vi "All-In-One_EIC-DIRC_DAQ_v3.vi"() -> ()   [LabVIEW 2024]
uses:
  C:/Users/hpDIRC/Desktop/eic_dirc_daq-LabVIEW_new/Thorlabs/Thorlabs.MotionControl.Controls.dll
  Thorlabs/Thorlabs.MotionControl.Controls.dll
  <vilib>/numeric/Random Number (Range) DBL.vi
  C:/Users/hpDIRC/Desktop/eic_dirc_daq-LabVIEW_new/Thorlabs/Thorlabs.MotionControl.IntegratedStepperMotorsCLI.dll
  Thorlabs/Thorlabs.MotionControl.IntegratedStepperMotorsCLI.dll
  C:/Users/hpDIRC/Desktop/eic_dirc_daq-LabVIEW_new/Thorlabs/Thorlabs.MotionControl.Benchtop.StepperMotorCLI.dll
  Thorlabs/Thorlabs.MotionControl.Benchtop.StepperMotorCLI.dll
panel:
  out "Just-Measure-Last":bool
  in  "Just Measure Length":dbl=100.0
  out "counter":dbl=184.0 caption="Measurements Recorded" format="%#_13g"
  in  "Just Measure":bool
  in  "alignment points":dbl=20.0 format="%#_13g"
  in  "BA step size":dbl=0.1 format="%#_13g"
  in  "BA3 BarY start":dbl=20.0 format="%#_13g"
  in  "BA3 BarX start":dbl=229.0 format="%#_13g"
  in  "BA2 BarY start":dbl=15.0 format="%#_13g"
  in  "BA2 BarX start":dbl=229.0 format="%#_13g"
  in  "BA PDA":dbl=180.0 format="%#_13g"
  in  "BA BMA":dbl=45.0 format="%#_13g"
  in  "BA PDY":dbl=126.0 format="%#_13g"
  in  "BA PDX":dbl=268.0 format="%#_13g"
  in  "BA1 Bar Y start":dbl=30.0 format="%#_13g"
  in  "BA1 BarX start":dbl=229.0 format="%#_13g"
  in  "# BA measurement points":i32=10
  in  "# IR measurement points":i32=10
  in  "IR step size":dbl=0.1 format="%#_13g"
  in  "IR3 BarY start":dbl=32.0 format="%#_13g"
  in  "IR3 BarX start":dbl=82.5 format="%#_13g"
  in  "IR2 BarY start":dbl=15.0 format="%#_13g"
  in  "IR2 BarX start":dbl=82.5 format="%#_13g"
  in  "PB PDA":dbl=180.0 format="%#_13g"
  in  "PB BMA":dbl=45.0 format="%#_13g"
  in  "PB PDY":dbl=126.0 format="%#_13g"
  in  "PB PDX":dbl=266.0 format="%#_13g"
  in  "IR PDA":dbl=238.0 format="%#_13g"
  in  "IR BMA":dbl=17.148 format="%#_13g"
  in  "IR PDY":dbl=119.5 format="%#_13g"
  in  "IR PDX":dbl=232.0 format="%#_13g"
  in  "PB Bar Y":dbl=30.0 format="%#_13g"
  in  "PB Bar X":dbl=170.0 format="%#_13g"
  in  "IR1 Bar Y start":dbl=20.0 format="%#_13g"
  in  "IR1 Bar X start":dbl=82.5 format="%#_13g"
  out "Ambient Temperature":dbl format="%#.2g"
  in  "bar-note":u16(ring) items=["Pure Beam (PB)", "Internal Reflection (IR)", "Bulk Attenuation (BA)"]
  out "meter-error":errorcluster
  out "NM-pts-tested":dbl caption="# Pts Tested for Alignment"
  in  "align-only":bool
  in  "run-BA":bool
  in  "run-IR":bool
  in  "PDY start":dbl=105.8
  in  "PDX start":dbl=265.0
  out "run time (min)":dbl
  out "alignment-counter":dbl=184.0 format="%#_13g"
  out "Optimized Location":dbl[](array[numeric])
  in  "Test Start Delay (s)":dbl=30.0
  out "queue-length":i32 caption="Queue Elements Remaining:"
  out "next-state-cluster-const":T1={"next-state"="", "bypass-confirm"=FALSE, "PDX"=300.0, "PDY"=150.0, "BarX"=300.0, "BarY"=150.0, "BMA"=45.0, "PDA"=85.0, "bar-note"=0, "meas#"=0}
  in  "X start":dbl=262.0
  in  "X end":dbl=263.0
  in  "Y end":dbl=121.5 format="%#_13g"
  in  "X step size":dbl=0.2 format="%#_13g"
  in  "Y step size":dbl=0.2
  in  "Y start":dbl=120.5 format="%#_13g"
  in  "centered-diode-scan":bool
  out "keep-file":bool
  out "main-stage-refs":T2
  out "state-queue":T3(array[cluster])
  out "loop-rate":u32
  out "meter-stat":bool caption="Log Status"
  out "stage-stat":bool caption="Log Status"
  out "Current Time:":string
  out "log-error":errorcluster
  out "log-path":path caption="Path Data Will Save To:"
  out "start-msg":string
  out "stage-error":errorcluster
  in  "PD Angle":refnum<k24>(container)
  in  "Brewster":refnum<k24>(container)
  in  "PD Y":refnum<k24>(container)
  in  "PD X":refnum<k24>(container)
  in  "BAR Y":refnum<k24>(container)
  in  "stop":bool
  in  "BAR X":refnum<k24>(container)
  out "pd-plt":cluster{"[0]":dbl, "[1]":dbl, "[2]":dbl}(graph) caption="Measurement History"
  out "pd3_v":dbl caption="PD 3" format="%#.4g"
  out "pd2_v":dbl caption="PD 2" format="%#.4g"
  out "pd1_v":dbl caption="PD 1" format="%#.4g"
  # "IR settings"
  # "°C"
  # "EXPERT DEBUGGING INFO"
  # "A"
  # "A"
  # "BA settings"
  # "A"
  # "Work In Progress - please do not use"
  # "Bar Note Readback:"
  # "PB settings"
  # "PD ONLY SCAN - CENTERED"
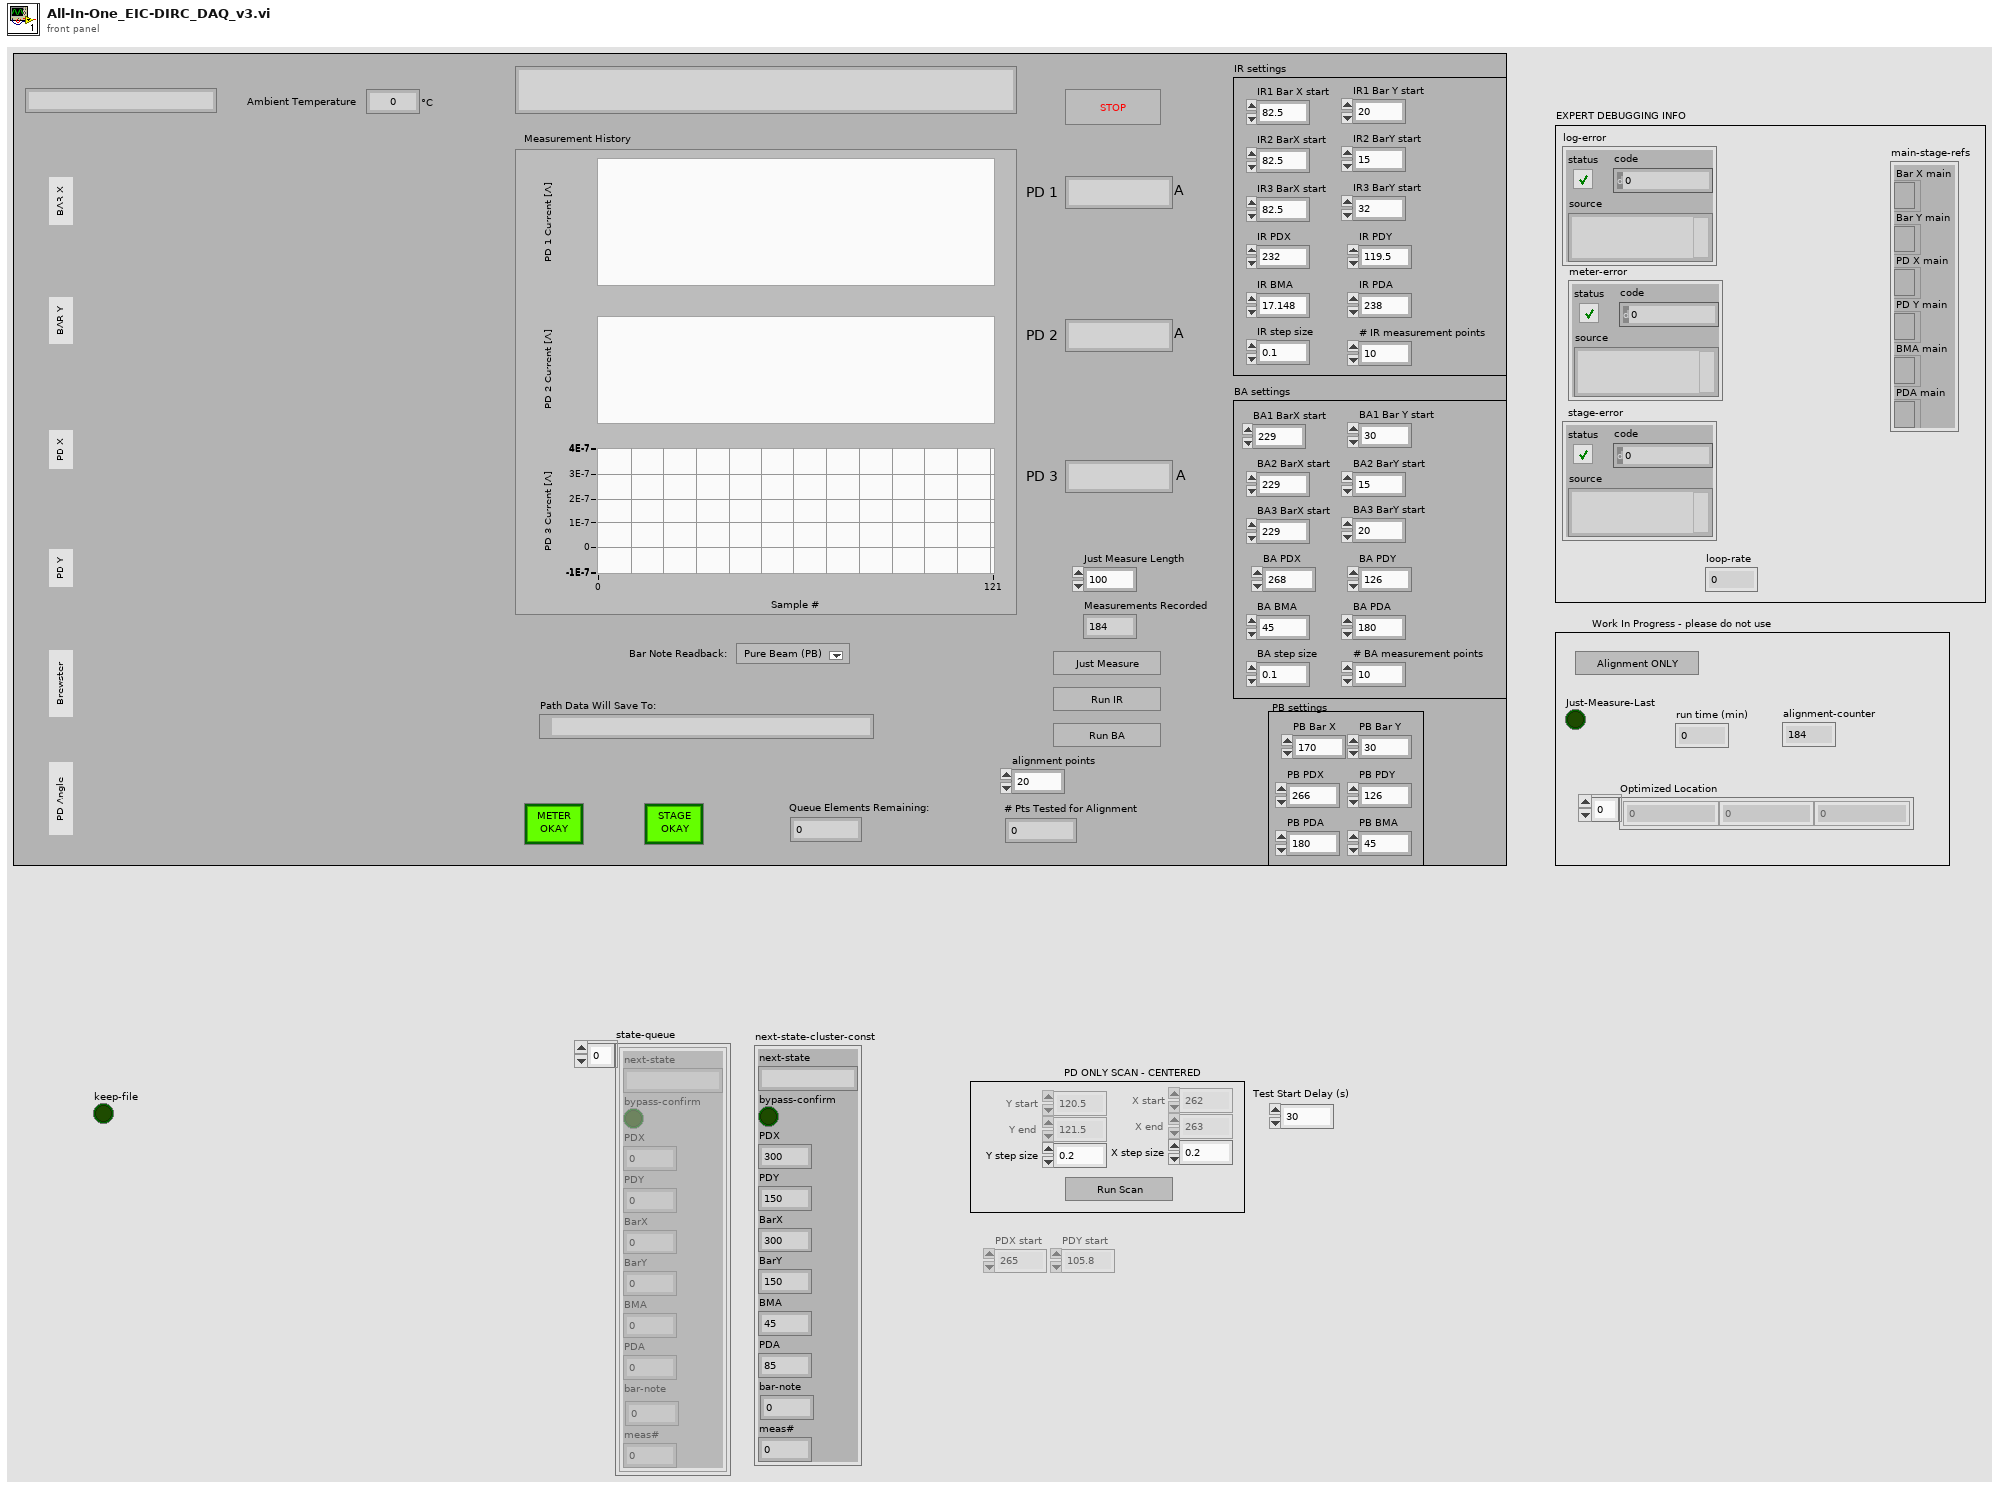
[diagram p1: front panel]
types:
  T1 = cluster{"next-state":string, "bypass-confirm":bool, "PDX":dbl, "PDY":dbl, "BarX":dbl, "BarY":dbl, "BMA":dbl, "PDA":dbl, "bar-note":u8, "meas#":u32}
  T2 = cluster{"Bar X main":refnum<k24>, "Bar Y main":refnum<k24>, "PD X main":refnum<k24>, "PD Y main":refnum<k24>, "BMA main":refnum<k24>, "PDA main":refnum<k24>}
  T3 = cluster{"next-state":string, "bypass-confirm":bool, "PDX":dbl, "PDY":dbl, "BarX":dbl, "BarY":dbl, "BMA":dbl, "PDA":dbl, "bar-note":u8, "meas#":u32}[]
  T4 = cluster{"Bar X":refnum<k24>, "Bar Y":refnum<k24>, "PD X":refnum<k24>, "PD Y":refnum<k24>, "Brewster":refnum<k24>, "PD Angle":refnum<k24>}
  T5 = enum16{"open", "replace", "create", "open or create", "replace or create", "replace or create with confirmation"}
  T6 = cluster{"alpha":dbl, "gamma":dbl, "rho":dbl, "sigma":dbl, "simplex L":dbl}
  T7 = cluster{"next-state":string, "mode-select":enum32{"IR", "Pure", "Bulk", "Bar Out", "stored-loc", "custom"}, "bypass-confirm":bool, "PDX":dbl, "PDY":dbl, "BarX":dbl, "BarY":dbl, "BMA":dbl, "PDA":dbl, "bar-note":bool}
  T8 = cluster{"[0]":dbl, "[1]":dbl, "[2]":dbl, "[3]":dbl, "[4]":dbl, "[5]":dbl, "[6]":dbl, "[7]":dbl, "[8]":dbl}
  T9 = cluster{"Bar X":dbl, "Bar Y":dbl, "PD X":dbl, "PD Y":dbl, "BMA":dbl, "PDA":dbl}
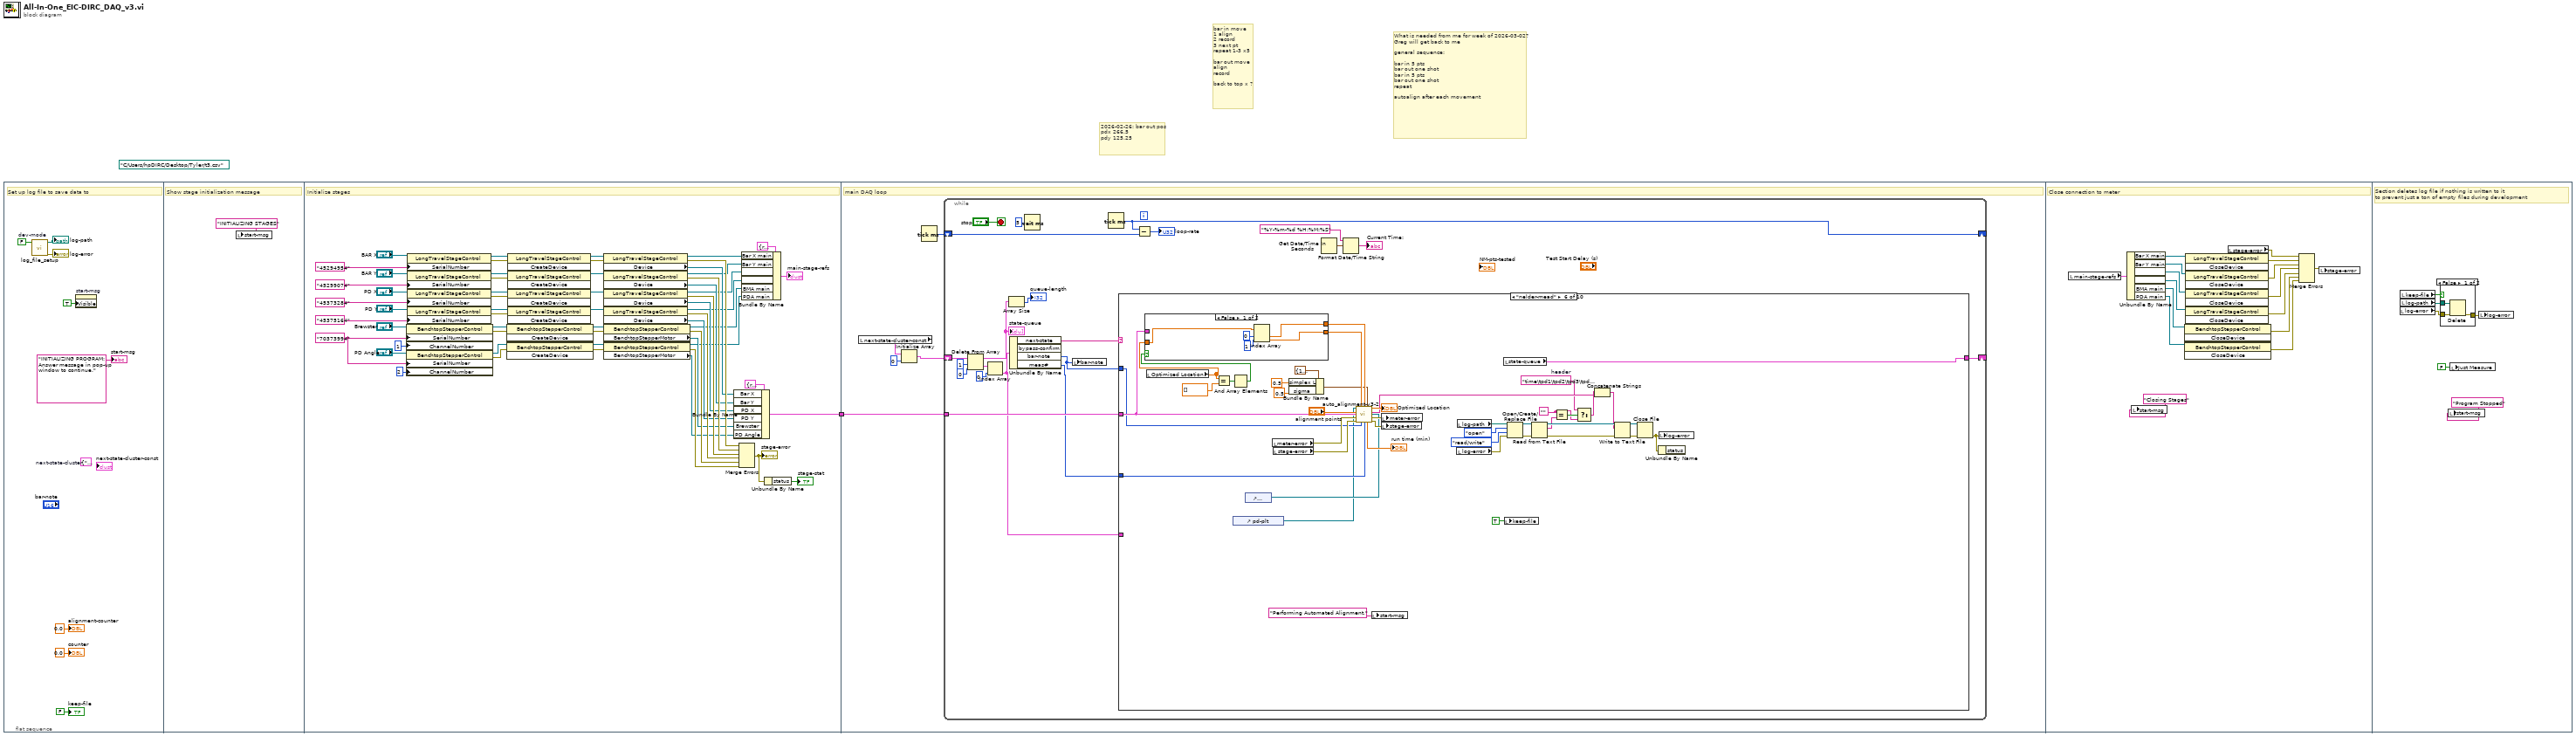
[diagram p0: block diagram]
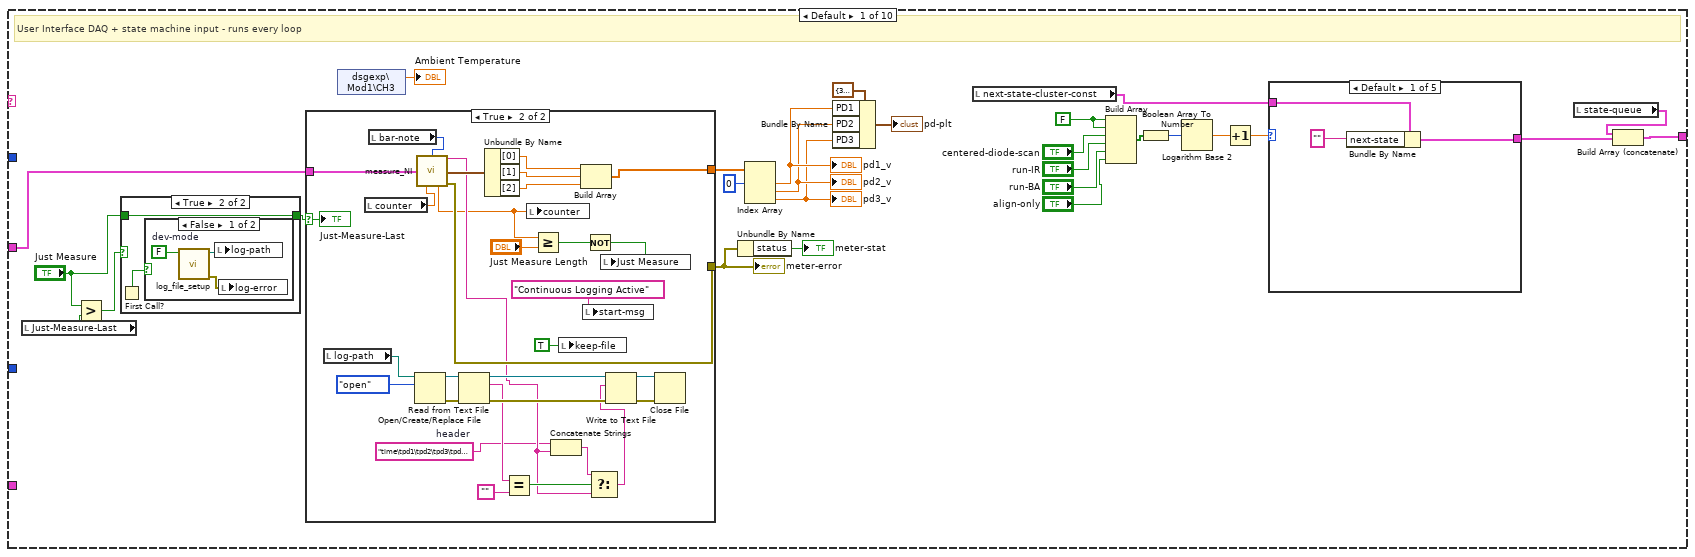
[diagram p2: hidden frame]
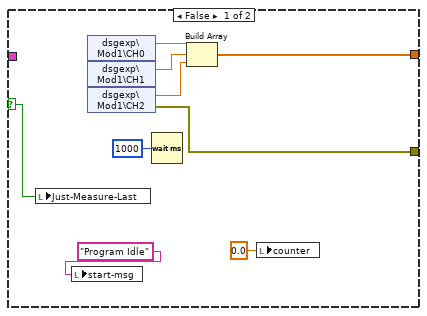
[diagram p5: hidden frame]
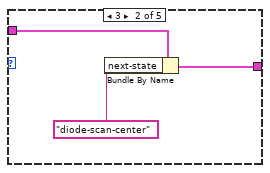
[diagram p6: hidden frame]
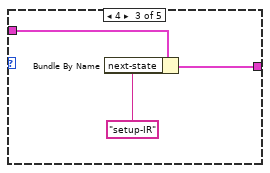
[diagram p7: hidden frame]
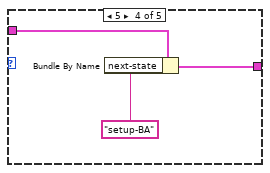
[diagram p8: hidden frame]
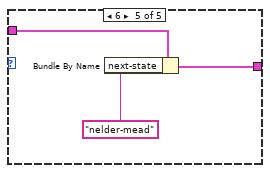
[diagram p9: hidden frame]
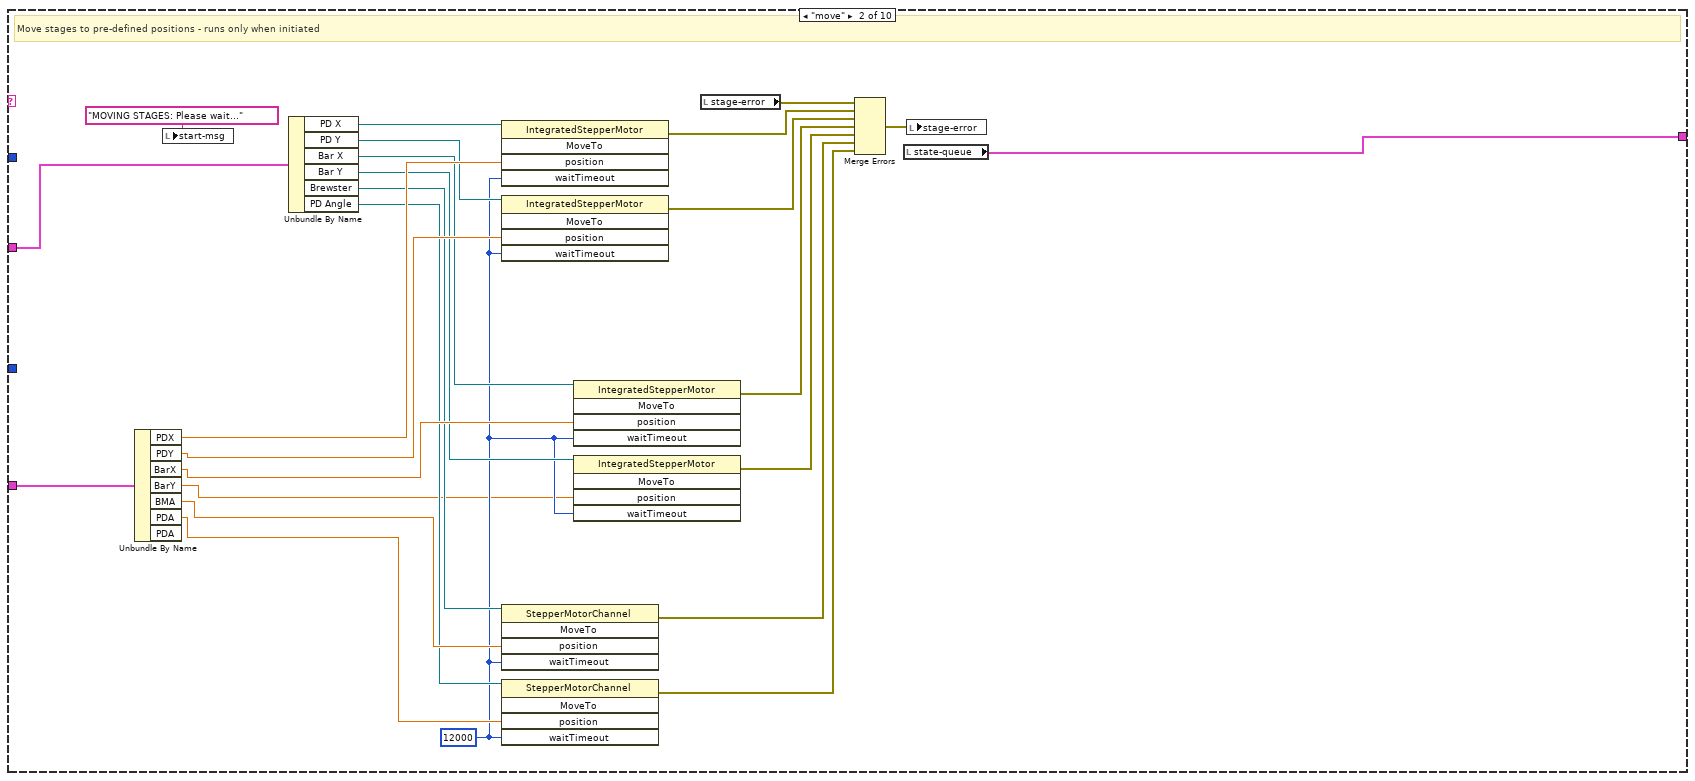
[diagram p10: hidden frame]
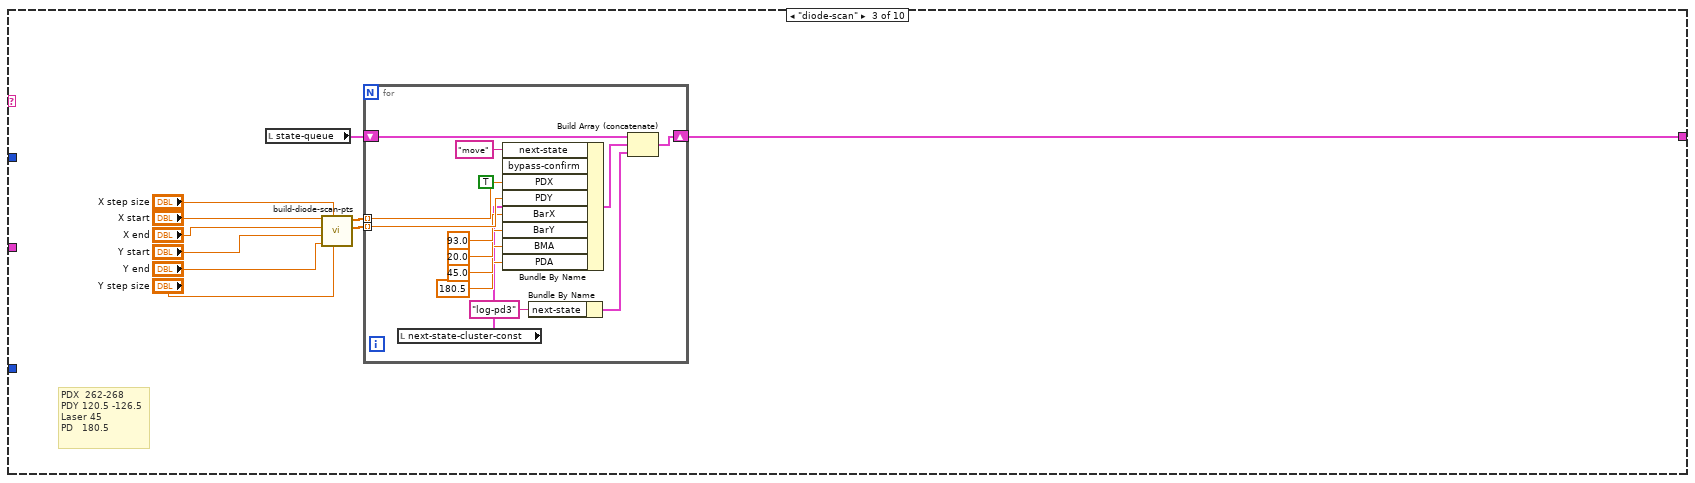
[diagram p11: hidden frame]
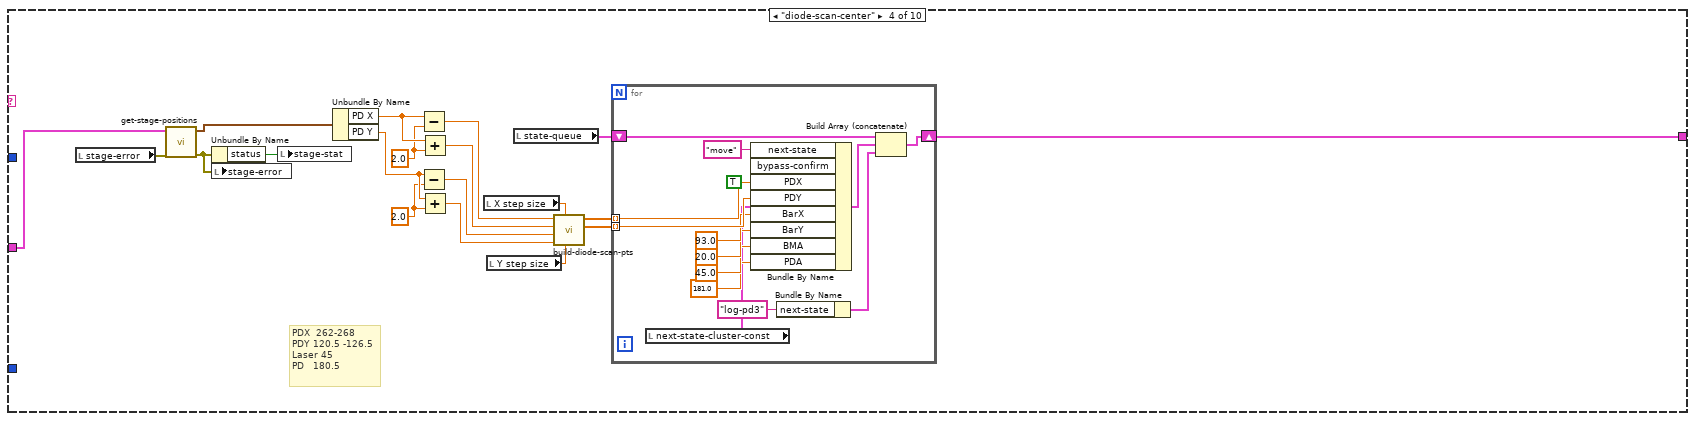
[diagram p12: hidden frame]
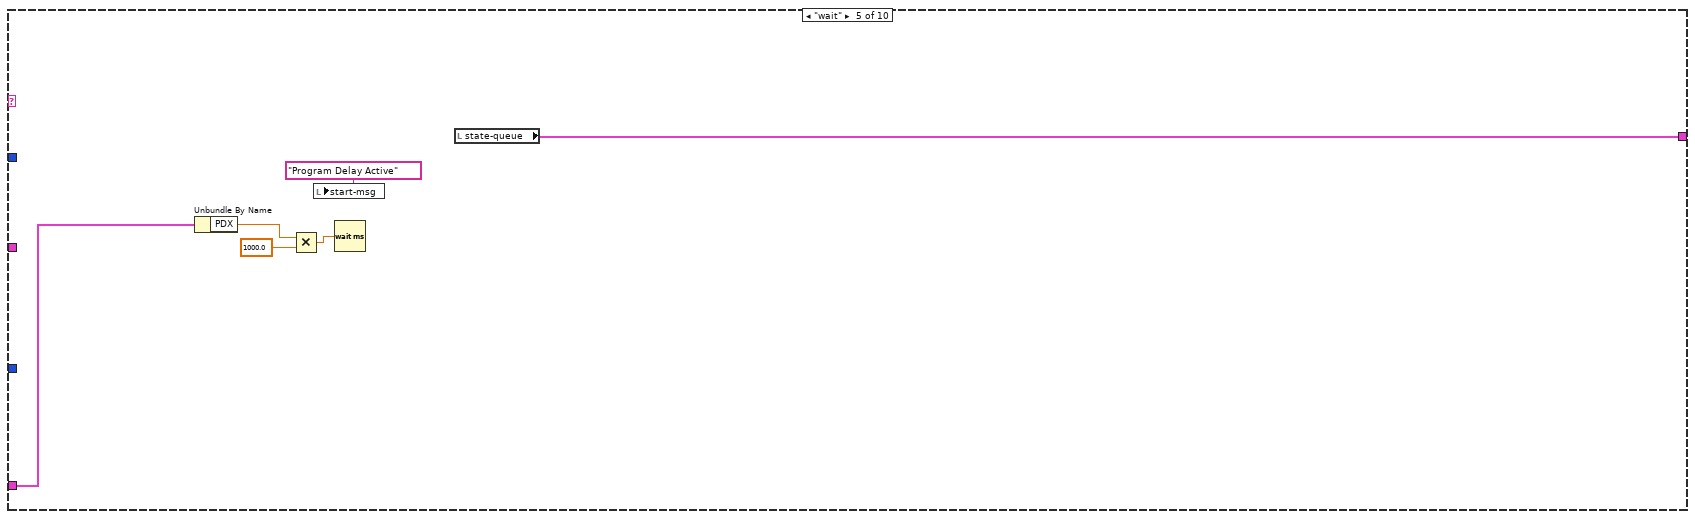
[diagram p13: hidden frame]
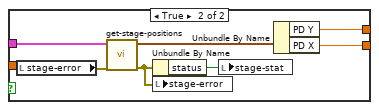
[diagram p14: hidden frame]
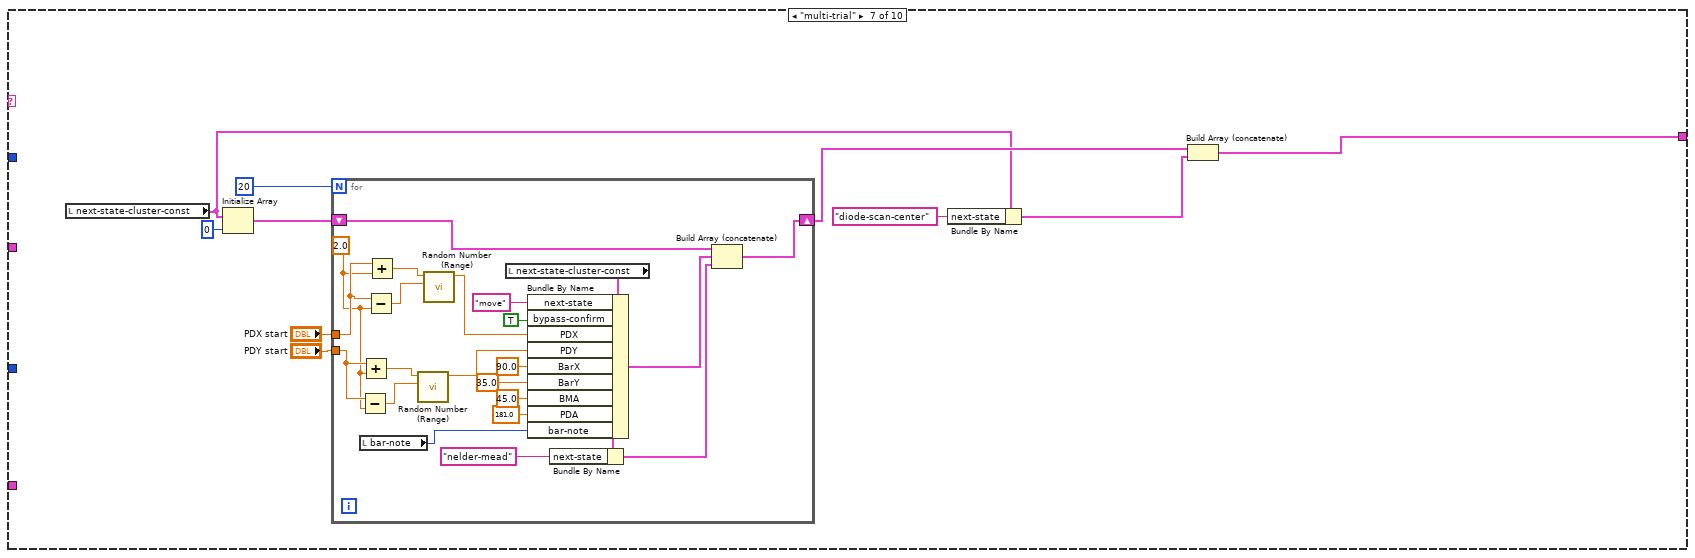
[diagram p15: hidden frame]
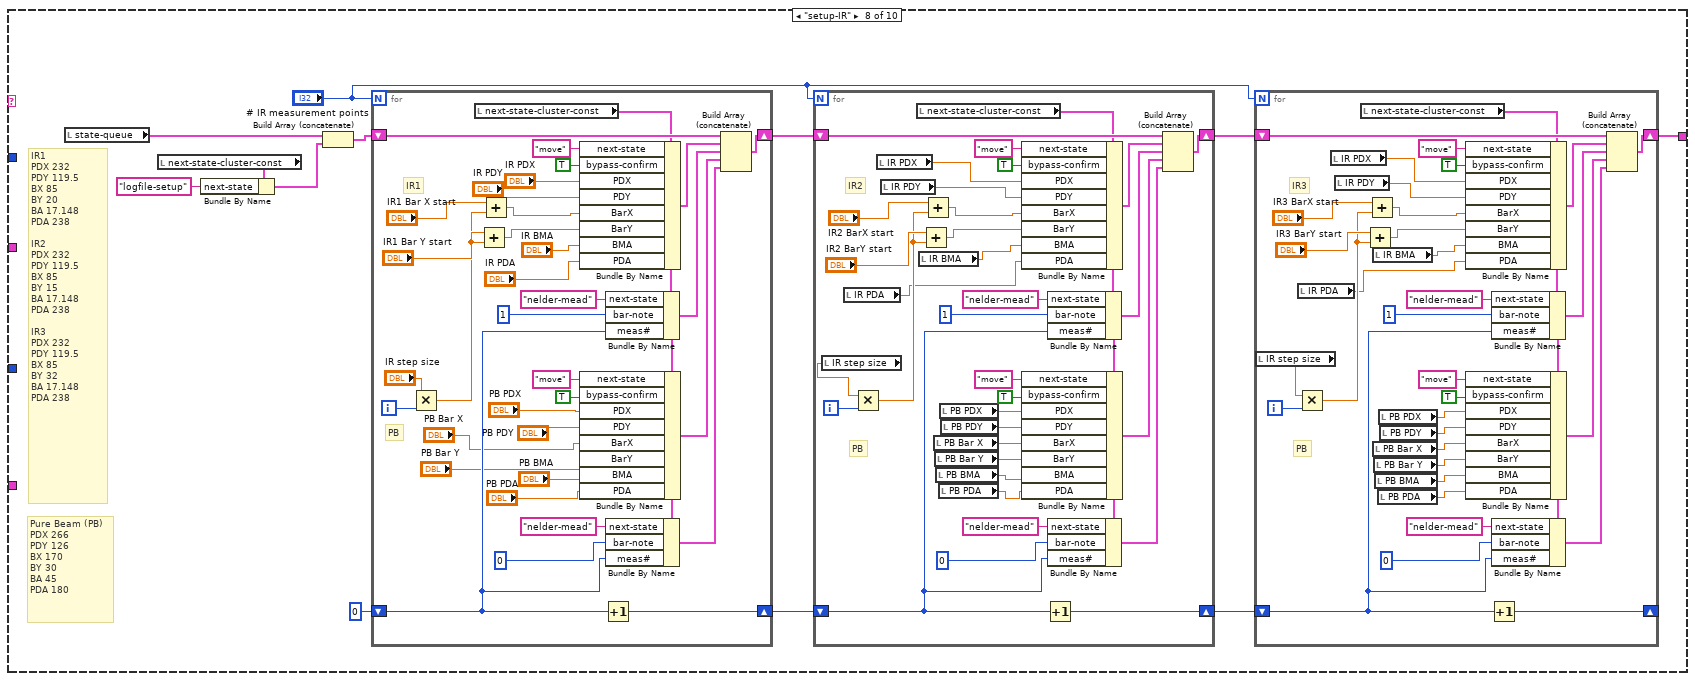
[diagram p16: hidden frame]
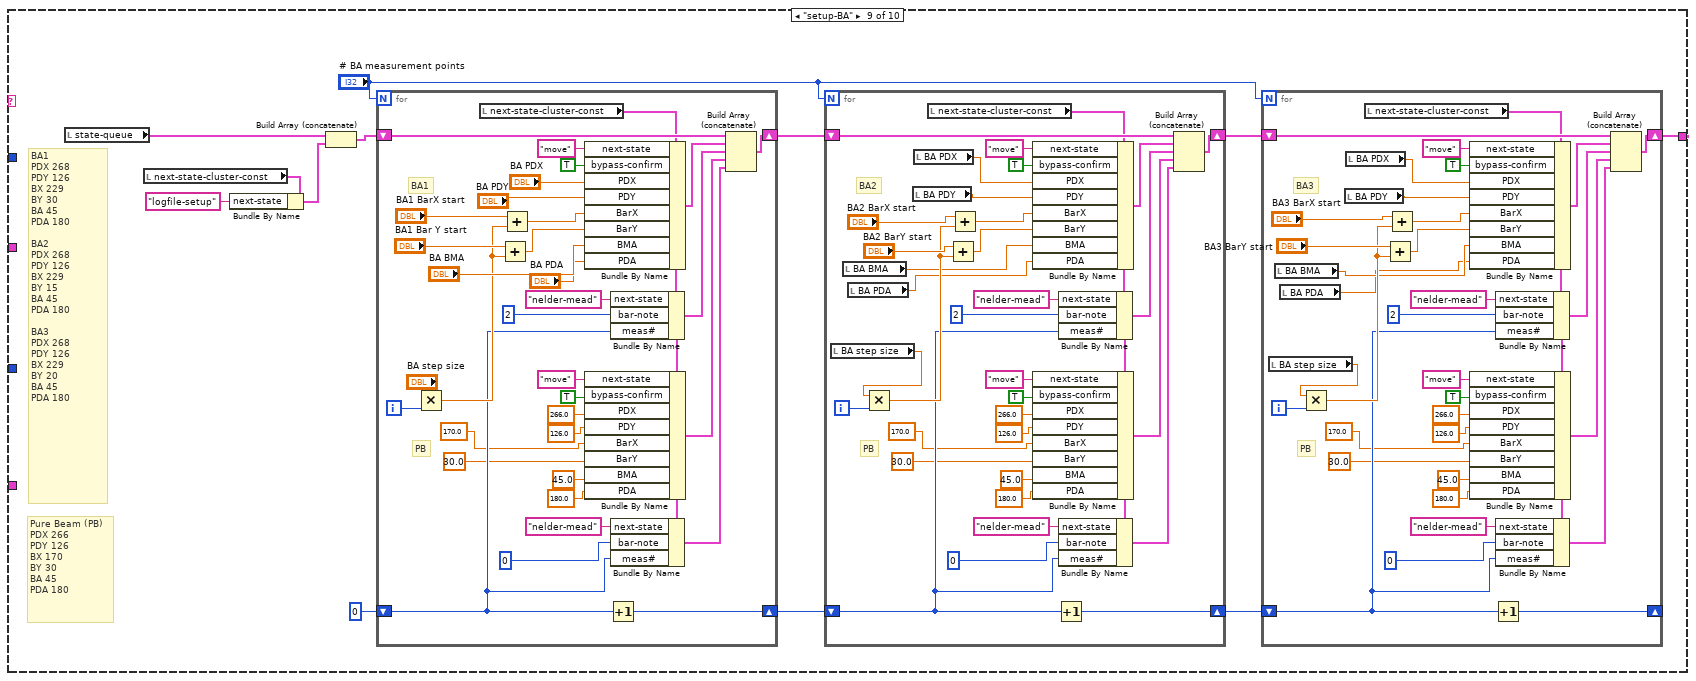
[diagram p17: hidden frame]
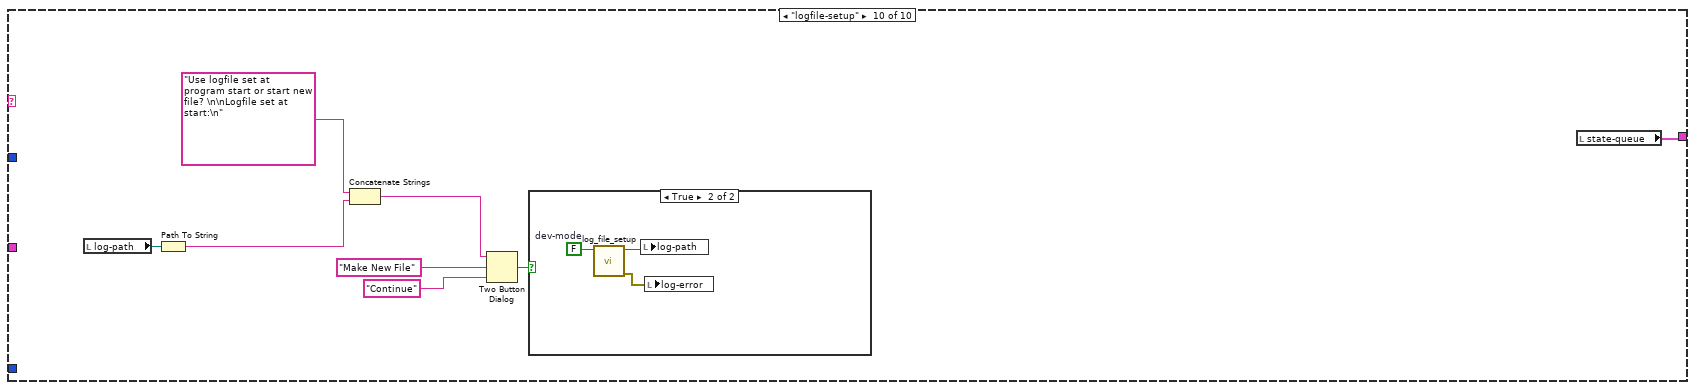
[diagram p18: hidden frame]
diagram:
  (unwired) path "C:/Users/hpDIRC/Desktop/Tyler/t3.csv" ("log-path")
  # "2026-02-26: bar out pos\npdx 266.5\npdy 125.25"
  # "bar in move\n1 align\n2 record\n3 next pt\nrepeat 1-3 x5\n\nbar out move\nalign\nrecord\n\nback to top x ?"
  # "What is needed from me for week of 2026-03-02?\nGreg will get back to me\n\ngeneral sequence:\n\nbar in 5 pts \nbar out one shot\nbar in 5 pts\nbar out one shot\nrepeat\n\nautoalign after each movement"
  n1 = flat-sequence {
    tunnel: [w21] -> w1
    tunnel: w1 -> [w72]
    frame #0 {
      w5 = FALSE  # dev-mode
      (unwired) T7 {"next-state"="", "mode-select"=enum."IR", "bypass-confirm"=FALSE, "PDX"=300.0, "PDY"=150.0, "BarX"=300.0, "BarY"=150.0, "BMA"=45.0, "PDA"=85.0, "bar-note"=FALSE}  # next-state-cluster
      # "Set up log file to save data to"
      n2 = call "log_file_setup.vi"("dev-mode"=w5) -> ("error out"=→"log-error":errorcluster, "appended path"=→"log-path":path)  [unwired: 8 in, 1 out]
      n3 = property on="start-msg" class="Str"("Visible"=TRUE) -> ()  [unwired: 2 in, 2 out]
      "start-msg" <- "INITIALIZING PROGRAM: Answer message in pop-up window to continue." ("String")
      "keep-file" <- FALSE
      "alignment-counter" <- 0.0 ("alignment-counter")
      "counter" <- 0.0 ("alignment-counter")
    }
    frame #1 {
      # "Show stage initialization message"
      n4 = local write "start-msg"("INITIALIZING STAGES" ("String")) -> ()
    }
    frame #2 {
      w28 = "70373994" ("SerialNumber")
      # "Initialize stages"
      n5 = property class="BenchtopStepperControl"(reference="Brewster", "SerialNumber"=w28, "ChannelNumber"=1) -> (reference out=w54:refnum<k24>, error out=w55:errorcluster)  [unwired: 1 in]
      n6 = property class="BenchtopStepperControl"(reference="PD Angle", "SerialNumber"=w28, "ChannelNumber"=2) -> (reference out=w53:refnum<k24>, error out=w56:errorcluster)  [unwired: 1 in]
      n7 = property class="LongTravelStageControl"(reference="BAR X", "SerialNumber"="45294954") -> (reference out=w31:refnum<k24>, error out=w38:errorcluster)  [unwired: 1 in]
      n8 = property class="LongTravelStageControl"(reference="BAR Y", "SerialNumber"="45299074") -> (reference out=w32:refnum<k24>, error out=w39:errorcluster)  [unwired: 1 in]
      n9 = property class="LongTravelStageControl"(reference="PD X", "SerialNumber"="45373284") -> (reference out=w35:refnum<k24>, error out=w40:errorcluster)  [unwired: 1 in]
      n10 = property class="LongTravelStageControl"(reference="PD Y", "SerialNumber"="45375164") -> (reference out=w36:refnum<k24>, error out=w41:errorcluster)  [unwired: 1 in]
      n11 = invoke class="BenchtopStepperControl" method="CreateDevice"(reference=w54, error in=w55) -> (reference out=w51:refnum<k24>, error out=w49:errorcluster)  [unwired: 1 in, 1 out]
      n12 = invoke class="BenchtopStepperControl" method="CreateDevice"(reference=w53, error in=w56) -> (reference out=w50:refnum<k24>, error out=w52:errorcluster)  [unwired: 1 in, 1 out]
      n13 = invoke class="LongTravelStageControl" method="CreateDevice"(reference=w31, error in=w38) -> (reference out=w44:refnum<k24>, error out=w48:errorcluster)  [unwired: 1 in, 1 out]
      n14 = invoke class="LongTravelStageControl" method="CreateDevice"(reference=w32, error in=w39) -> (reference out=w45:refnum<k24>)  [unwired: 1 in, 2 out]
      n15 = invoke class="LongTravelStageControl" method="CreateDevice"(reference=w35, error in=w40) -> (reference out=w46:refnum<k24>)  [unwired: 1 in, 2 out]
      n16 = invoke class="LongTravelStageControl" method="CreateDevice"(reference=w36, error in=w41) -> (reference out=w47:refnum<k24>)  [unwired: 1 in, 2 out]
      n17 = property class="BenchtopStepperControl"(reference=w51, error in=w49) -> (reference out=w15:refnum<k24>, error out=w66:errorcluster, "BenchtopStepperMotor"=w61:refnum<k24>)
      n18 = property class="BenchtopStepperControl"(reference=w50, error in=w52) -> (reference out=w14:refnum<k24>, error out=w67:errorcluster, "BenchtopStepperMotor"=w62:refnum<k24>)
      n19 = property class="LongTravelStageControl"(reference=w44, error in=w48) -> (reference out=w19:refnum<k24>, error out=w68:errorcluster, "Device"=w57:refnum<k24>)
      n20 = property class="LongTravelStageControl"(reference=w45) -> (reference out=w18:refnum<k24>, error out=w63:errorcluster, "Device"=w58:refnum<k24>)  [unwired: 1 in]
      n21 = property class="LongTravelStageControl"(reference=w46) -> (reference out=w17:refnum<k24>, error out=w64:errorcluster, "Device"=w59:refnum<k24>)  [unwired: 1 in]
      n22 = property class="LongTravelStageControl"(reference=w47) -> (reference out=w16:refnum<k24>, error out=w65:errorcluster, "Device"=w60:refnum<k24>)  [unwired: 1 in]
      n23 = Bundle By Name(cluster=T4 {"Bar X"=refnum, "Bar Y"=refnum, "PD X"=refnum, "PD Y"=refnum, "Brewster"=refnum, "PD Angle"=refnum}, "Bar X"=w57, "Bar Y"=w58, "PD X"=w59, "PD Y"=w60, "Brewster"=w61, "PD Angle"=w62) -> (w21:T4)
      n24 = Merge Errors(w68, w63, w64, w65, w66, w67) -> (w12:errorcluster)
      "stage-error" <- w12
      n25 = Bundle By Name(cluster=T2 {"Bar X main"=refnum, "Bar Y main"=refnum, "PD X main"=refnum, "PD Y main"=refnum, "BMA main"=refnum, "PDA main"=refnum}, "Bar X main"=w19, "Bar Y main"=w18, "PD X main"=w17, "PD Y main"=w16, "BMA main"=w15, "PDA main"=w14) -> (→"main-stage-refs":T2)
      n26 = Unbundle By Name(w12) -> ("status"=→"stage-stat":bool)
    }
    frame #3 {
      # "main DAQ loop"
      n27 = local read "next-state-cluster-const"() -> (w69:T1)
      n28 = Initialize Array(w69, 0 ("dimension size")) -> (w71:T3)
      n29 = Tick Count (ms)() -> (millisecond timer value=w73:u32)
      n30 = while {
        shift-right: [w93] -> _
        shift-left: w73 -> [w92]
        tunnel: w72 -> [w90]
        shift-right: [w79] -> _
        shift-left: w71 -> [w81]
        stop <- "stop" stop-if-true
        n31 = Delete From Array(array=w81, length=1, index=0) -> (deleted portion=w80:T3, array with subset deleted=w77:T3)
        "state-queue" <- w77
        n32 = Index Array(array=w80, index=0) -> (element=w78:T1)
        n33 = Array Size(array=w77) -> (size(s)=→"queue-length":i32)
        n34 = Unbundle By Name(w78) -> ("next-state"=w82:string, "bar-note"=w76:u8, "meas#"=w75:u32)  [unwired: 1 out]
        n35 = Wait (ms)(milliseconds to wait=u32 5) -> ()  [unwired: 1 out]
        n36 = local write "bar-note"(w76) -> ()
        n37 = Tick Count (ms)() -> (millisecond timer value=w93:u32)
        n38 = case shown="\"nelder-mead\"" w82 {
          tunnel: w90 -> [w101 w210 _ w243 _ w302 _ _ _ _]
          tunnel: [w113 w209 w217 w250 w269 w316 w331 w366 w480 w596] -> w79
          tunnel: w78 -> [_ w207 _ _ w270 _ _ _ _ _]
          tunnel: w76 -> [_ _ _ _ _ w301 _ _ _ _]
          tunnel: w75 -> [_ _ _ _ _ w300 _ _ _ _]
          frame Default {
            w102 = FALSE ("element")
            # "User Interface DAQ + state machine input - runs every loop"
            n39 = local read "Just-Measure-Last"() -> (w98:bool)
            n40 = Greater?(x="Just Measure", y=w98) -> (0:w97:bool)
            n41 = case shown="True" w97 {
              tunnel: "Just Measure" -> [w123 w125]
              tunnel: [w123 w125] -> w95
              frame False {
              }
              frame True {
                n42 = First Call?() -> (First Call?: T/F=w124:bool)
                n43 = case shown="False" w124 {
                  frame False {
                    w126 = FALSE  # dev-mode
                    n44 = call "log_file_setup.vi"("dev-mode"=w126) -> ("error out"=w127:errorcluster, "appended path"=w128:path)  [unwired: 8 in, 1 out]
                    n45 = local write "log-path"(w128) -> ()
                    n46 = local write "log-error"(w127) -> ()
                  }
                  frame True {
                  }
                }
              }
            }
            n47 = case shown="True" w95 {
              selector: w95 -> [w130 w141]
              tunnel: [w139 w163] -> w103
              tunnel: w101 -> [_ w170]
              tunnel: [w132 w168] -> w99
              frame False {
                n48 = local write "Just-Measure-Last"(w130) -> ()
                n49 = local write "start-msg"("Program Idle" ("String")) -> ()
                n50 = shared-variable "dsgexp\\Mod1\\CH0"() -> (w138:dbl, error out=w135:errorcluster)  [unwired: 1 in]
                n51 = shared-variable "dsgexp\\Mod1\\CH1"(error in=w135) -> (w137:dbl, error out=w134:errorcluster)
                n52 = shared-variable "dsgexp\\Mod1\\CH2"(error in=w134) -> (w136:dbl, error out=w132:errorcluster)
                n53 = Wait (ms)(milliseconds to wait=u32 1000) -> ()  [unwired: 1 out]
                n54 = Build Array(w138, w137, w136) -> (w139:dbl[])
                n55 = local write "counter"(0.0 ("counter")) -> ()
              }
              frame True {
                w148 = "time\tpd1\tpd2\tpd3\tpd3/pd1\tpd2/pd1\tbx\tby\tpdx\tpdy\tpda\tbm\tbar-note\tmeas#\tpt#\n"  # header
                n56 = local read "log-path"() -> (w161:path)
                n57 = local read "counter"() -> (w162:dbl)
                n58 = local read "bar-note"() -> (w169:u16)
                n59 = Open/Create/Replace File(file path (use dialog)=w161, operation (0:open)=T5."open") -> (refnum out=w158:refnum<file>, error out=w159:errorcluster)  [unwired: 4 in, 1 out]
                n60 = call "measure_NI.vi"("bar-note"=w169, "stage-refs"=w170, "counter-in"=w162) -> ("logfile-line-out"=w149:string, "PD out"=w167:T8, "counter-out"=w145:dbl, "stage-error-out"=w168:errorcluster)  [unwired: 7 in, 2 out]
                n61 = Read from Text File(file (use dialog)=w158, error in=w159) -> (refnum out=w156:refnum<file>, text=w151:string, error out=w157:errorcluster)  [unwired: 2 in, 1 out]
                n62 = Unbundle By Name(w167) -> ("[0]"=w166:dbl, "[1]"=w165:dbl, "[2]"=w164:dbl)
                n63 = Equal?(x=w151, y="") -> (x = y?=w150:bool)
                n64 = local write "counter"(w145) -> ()
                n65 = Greater Or Equal?(x=w145, y="Just Measure Length") -> (x >= y?=w143:bool)
                n66 = Concatenate Strings(w148, w149) -> (w147:string)
                n67 = local write "keep-file"(TRUE ("keep-file")) -> ()
                n68 = Build Array(w166, w165, w164) -> (w163:dbl[])
                n69 = local write "start-msg"("Continuous Logging Active" ("String")) -> ()
                n70 = Not(x=w143) -> (.not. x?=w142:bool)
                n71 = Select(t=w147, s=w150, f=w149) -> (s? t:f=w146:string)
                n72 = local write "Just Measure"(w142) -> ()
                n73 = Write to Text File(file (use dialog)=w156, text=w146, error in=w157) -> (refnum out=w154:refnum<file>, error out=w155:errorcluster)  [unwired: 1 in, 1 out]
                n74 = Close File(refnum=w154, error in=w155) -> ()  [unwired: 2 out]
                "Just-Measure-Last" <- w141
              }
            }
            "meter-error" <- w99
            n75 = shared-variable "dsgexp\\Mod1\\CH3"() -> (→"Ambient Temperature":dbl)  [unwired: 1 in, 1 out]
            n76 = Unbundle By Name(w99) -> ("status"=→"meter-stat":bool)
            n77 = Index Array(array=w103, index #1=0 ("index")) -> (element #1=w120:dbl, element #2=w119:dbl, element #3=w118:dbl)  [unwired: 2 in]
            "pd3_v" <- w118
            "pd2_v" <- w119
            "pd1_v" <- w120
            n78 = Bundle By Name(cluster=cluster{"PD1":dbl, "PD2":dbl, "PD3":dbl} {"PD1"=3e-05, "PD2"=3e-05, "PD3"=3e-05} ("PD ranges"), "PD1"=w120, "PD2"=w119, "PD3"=w118) -> (→"pd-plt":cluster{"PD1":dbl, "PD2":dbl, "PD3":dbl})
            n79 = local read "next-state-cluster-const"() -> (w111:T1)
            n80 = Build Array(w102, w102, "centered-diode-scan", "run-IR", "run-BA", "align-only") -> (w116:bool[])
            n81 = Boolean Array To Number(Boolean array=w116) -> (number=w108:u32)
            n82 = Logarithm Base 2(1:w108) -> (0:w110:dbl)
            n83 = Increment(x=w110) -> (x+1=w109:dbl)
            n84 = case shown="Default" w109 {
              tunnel: w111 -> [w173 w176 w179 w182 w185]
              tunnel: [w171 w174 w177 w180 w183] -> w112
              frame Default {
                n85 = Bundle By Name(cluster=w173, "next-state"="") -> (w171:T1)
              }
              frame 3 {
                n86 = Bundle By Name(cluster=w176, "next-state"="diode-scan-center") -> (w174:T1)
              }
              frame 4 {
                n87 = Bundle By Name(cluster=w179, "next-state"="setup-IR") -> (w177:T1)
              }
              frame 5 {
                n88 = Bundle By Name(cluster=w182, "next-state"="setup-BA") -> (w180:T1)
              }
              frame 6 {
                n89 = Bundle By Name(cluster=w185, "next-state"="nelder-mead") -> (w183:T1)
              }
            }
            n90 = local read "state-queue"() -> (w114:T3)
            n91 = Build Array (concatenate)(w114, w112) -> (w113:T3)
          }
          frame "move" {
            w187 = 12000 ("waitTimeout")
            # "Move stages to pre-defined positions - runs only when initiated"
            n92 = Unbundle By Name(w207) -> ("PDX"=w206:dbl, "PDY"=w205:dbl, "BarX"=w204:dbl, "BarY"=w186:dbl, "BMA"=w203:dbl, "PDA"=w202:dbl)  [unwired: 1 out]
            n93 = local write "start-msg"("MOVING STAGES: Please wait..." ("String")) -> ()
            n94 = Unbundle By Name(w210) -> ("PD X"=w193:refnum<k24>, "PD Y"=w188:refnum<k24>, "Bar X"=w189:refnum<k24>, "Bar Y"=w190:refnum<k24>, "Brewster"=w191:refnum<k24>, "PD Angle"=w192:refnum<k24>)
            n95 = invoke class="IntegratedStepperMotor" method="MoveTo"(reference=w193, "position"=w206, "waitTimeout"=w187) -> (error out=w200:errorcluster)  [unwired: 2 in, 4 out]
            n96 = invoke class="IntegratedStepperMotor" method="MoveTo"(reference=w188, "position"=w205, "waitTimeout"=w187) -> (error out=w199:errorcluster)  [unwired: 2 in, 4 out]
            n97 = invoke class="StepperMotorChannel" method="MoveTo"(reference=w191, "position"=w203, "waitTimeout"=w187) -> (error out=w196:errorcluster)  [unwired: 2 in, 4 out]
            n98 = invoke class="StepperMotorChannel" method="MoveTo"(reference=w192, "position"=w202, "waitTimeout"=w187) -> (error out=w195:errorcluster)  [unwired: 2 in, 4 out]
            n99 = invoke class="IntegratedStepperMotor" method="MoveTo"(reference=w189, "position"=w204, "waitTimeout"=w187) -> (error out=w198:errorcluster)  [unwired: 2 in, 4 out]
            n100 = invoke class="IntegratedStepperMotor" method="MoveTo"(reference=w190, "position"=w186, "waitTimeout"=w187) -> (error out=w197:errorcluster)  [unwired: 2 in, 4 out]
            n101 = local read "stage-error"() -> (w201:errorcluster)
            n102 = Merge Errors(w201, w200, w199, w198, w197, w196, w195) -> (w194:errorcluster)
            n103 = local read "state-queue"() -> (w209:T3)
            n104 = local write "stage-error"(w194) -> ()
          }
          frame "diode-scan" {
            # "PDX  262-268\nPDY 120.5 -126.5\nLaser 45\nPD   180.5"
            n105 = local read "state-queue"() -> (w220:T3)
            n106 = call "build-diode-scan-pts.vi"("Y step size"="Y step size", "X step size"="X step size", "Y end"="Y end", "Y start"="Y start", "X end"="X end", "X start"="X start") -> ("y"=w218:dbl[], "x"=w219:dbl[])  [unwired: 4 in]
            n107 = for {
              tunnel: w219 -> [w234] mode=indexing
              tunnel: w218 -> [w233] mode=indexing
              shift-right: [w227] -> w217
              shift-left: w220 -> [w229]
              n108 = local read "next-state-cluster-const"() -> (w221:T1)
              n109 = Bundle By Name(cluster=w221, "next-state"="move", "bypass-confirm"=TRUE, "PDX"=w234, "PDY"=w233, "BarX"=93.0, "BarY"=20.0, "BMA"=45.0, "PDA"=180.5) -> (w228:T1)
              n110 = Bundle By Name(cluster=w221, "next-state"="log-pd3") -> (w222:T1)
              n111 = Build Array (concatenate)(w229, w228, w222) -> (w227:T3)
            }
          }
          frame "diode-scan-center" {
            w238 = 2.0 ("y")
            w237 = 2.0 ("y")
            # "PDX  262-268\nPDY 120.5 -126.5\nLaser 45\nPD   180.5"
            n112 = local read "stage-error"() -> (w246:errorcluster)
            n113 = call "get-stage-positions.vi"("error in (no error)"=w246, "Cluster"=w243) -> ("error out"=w245:errorcluster, "stage positions"=w244:T9)  [unwired: 8 in]
            n114 = Unbundle By Name(w245) -> ("status"=w247:bool)
            n115 = local write "stage-error"(w245) -> ()
            n116 = local write "stage-stat"(w247) -> ()
            n117 = Unbundle By Name(w244) -> ("PD X"=w242:dbl, "PD Y"=w239:dbl)
            n118 = Subtract(x=w242, y=w237) -> (x-y=w241:dbl)
            n119 = Subtract(x=w239, y=w238) -> (x-y=w236:dbl)
            n120 = Add(x=w242, y=w237) -> (x+y=w240:dbl)
            n121 = Add(x=w239, y=w238) -> (x+y=w235:dbl)
            n122 = local read "X step size"() -> (w249:dbl)
            n123 = local read "Y step size"() -> (w248:dbl)
            n124 = local read "state-queue"() -> (w253:T3)
            n125 = call "build-diode-scan-pts.vi"("Y step size"=w248, "X step size"=w249, "Y end"=w235, "Y start"=w236, "X end"=w240, "X start"=w241) -> ("y"=w251:dbl[], "x"=w252:dbl[])  [unwired: 4 in]
            n126 = for {
              tunnel: w252 -> [w267] mode=indexing
              tunnel: w251 -> [w266] mode=indexing
              shift-right: [w260] -> w250
              shift-left: w253 -> [w262]
              n127 = local read "next-state-cluster-const"() -> (w254:T1)
              n128 = Bundle By Name(cluster=w254, "next-state"="move", "bypass-confirm"=TRUE, "PDX"=w267, "PDY"=w266, "BarX"=93.0, "BarY"=20.0, "BMA"=45.0, "PDA"=181.0) -> (w261:T1)
              n129 = Bundle By Name(cluster=w254, "next-state"="log-pd3") -> (w255:T1)
              n130 = Build Array (concatenate)(w262, w261, w255) -> (w260:T3)
            }
          }
          frame "wait" {
            n131 = Unbundle By Name(w270) -> ("PDX"=w271:dbl)
            n132 = Multiply(x=w271, y=1000.0) -> (x*y=w273:dbl)
            n133 = local write "start-msg"("Program Delay Active" ("String")) -> ()
            n134 = Wait (ms)(milliseconds to wait=w273) -> ()  [unwired: 1 out]
            n135 = local read "state-queue"() -> (w269:T3)
          }
          frame "nelder-mead" {
            w282 = "time\tpd1\tpd2\tpd3\tpd3/pd1\tpd2/pd1\tbx\tby\tpdx\tpdy\tpda\tbm\tbar-note\tmeas#\tpt#\n"  # header
            w286 = ""
            n136 = local read "Optimized Location"() -> (w274:dbl[])
            n137 = Equal?(x=w274, y=dbl[] [] ("Optimized Location 2")) -> (x = y?=w277:bool[])
            n138 = And Array Elements(Boolean array=w277) -> (logical AND=w275:bool)
            n139 = case shown="False" w275 {
              tunnel: [w318 w324] -> w313
              tunnel: [w319 w323] -> w312
              tunnel: w302 -> [_ w322]
              tunnel: w274 -> [w317 _]
              frame False {
                n140 = Index Array(array=w317, index #1=0 ("index"), index #2=1 ("index")) -> (element #1=w319:dbl, element #2=w318:dbl)
              }
              frame True {
                n141 = local read "stage-error"() -> (w327:errorcluster)
                n142 = call "get-stage-positions.vi"("error in (no error)"=w327, "Cluster"=w322) -> ("error out"=w326:errorcluster, "stage positions"=w325:T9)  [unwired: 8 in]
                n143 = Unbundle By Name(w326) -> ("status"=w328:bool)
                n144 = local write "stage-error"(w326) -> ()
                n145 = local write "stage-stat"(w328) -> ()
                n146 = Unbundle By Name(w325) -> ("PD Y"=w323:dbl, "PD X"=w324:dbl)
              }
            }
            n147 = control-ref of="pd-plt"() -> (w278:refnum<vi>)
            n148 = control-ref of="NM-pts-tested"() -> (w280:refnum<vi>)
            n149 = local read "meter-error"() -> (w315:errorcluster)
            n150 = local read "stage-error"() -> (w314:errorcluster)
            n151 = Bundle By Name(cluster=T6 {"alpha"=1.0, "gamma"=2.0, "rho"=0.5, "sigma"=0.5, "simplex L"=0.5} ("NM-params"), "simplex L"=0.5, "sigma"=0.5) -> (w305:T6)
            n152 = call "auto_alignment-v3-2.vi"("pd-plt"=w278, "xStart"=w313, "yStart"=w312, "NM-params"=w305, "alignmnet points"="alignment points", "stage-refs"=w302, "nPts"=w280, "meter-error"=w315, "stage-error"=w314, "bar-note"=w301, "meas#"=w300) -> ("Optimized Location"=→"Optimized Location":dbl[], "logfile-line-out"=w283:string, "meter-error-out"=w311:errorcluster, "run time (s)"=→"run time (min)":dbl, "stage-error-out"=w310:errorcluster)
            n153 = local write "start-msg"("Performing Automated Alignment." ("String")) -> ()
            n154 = local write "meter-error"(w311) -> ()
            n155 = local write "stage-error"(w310) -> ()
            n156 = local read "log-error"() -> (w298:errorcluster)
            n157 = local read "log-path"() -> (w299:path)
            n158 = local read "state-queue"() -> (w316:T3)
            n159 = local write "keep-file"(TRUE ("keep-file")) -> ()
            n160 = Open/Create/Replace File(file path (use dialog)=w299, error in=w298, operation (0:open)=T5."open", access (0:read/write)=enum16{"read/write", "read-only", "write-only"}."read/write") -> (refnum out=w297:refnum<file>, error out=w293:errorcluster)  [unwired: 2 in, 1 out]
            n161 = Read from Text File(file (use dialog)=w297, error in=w293) -> (refnum out=w294:refnum<file>, text=w290:string, error out=w292:errorcluster)  [unwired: 2 in, 1 out]
            n162 = Equal?(x=w286, y=w290) -> (x = y?=w289:bool)
            n163 = Select(t=w282, s=w289, f=w286) -> (s? t:f=w287:string)
            n164 = Concatenate Strings(w287, w283) -> (w288:string)
            n165 = Write to Text File(file (use dialog)=w294, text=w288, error in=w292) -> (refnum out=w296:refnum<file>, error out=w295:errorcluster)  [unwired: 1 in, 1 out]
            n166 = Close File(refnum=w296, error in=w295) -> (error out=w291:errorcluster)  [unwired: 1 out]
            n167 = Unbundle By Name(w291) -> ()  [unwired: 1 out]
            n168 = local write "log-error"(w291) -> ()
          }
          frame "multi-trial" {
            n169 = local read "next-state-cluster-const"() -> (w329:T1)
            n170 = Initialize Array(w329, 0 ("dimension size")) -> (w337:T3)
            n171 = for {
              N: 20 -> [_]
              shift-right: [w358] -> w332
              shift-left: w337 -> [w359]
              tunnel: "PDX start" -> [w346]
              tunnel: "PDY start" -> [w342]
              w341 = 2.0
              n172 = Subtract(x=w342, y=w341) -> (x-y=w343:dbl)
              n173 = local read "bar-note"() -> (w339:u16)
              n174 = Add(x=w342, y=w341) -> (x+y=w344:dbl)
              n175 = Subtract(x=w346, y=w341) -> (x-y=w348:dbl)
              n176 = Add(x=w346, y=w341) -> (x+y=w347:dbl)
              n177 = call-poly <vilib>:"Random Number (Range).vi"("lower bound (0)"=w343, "upper bound (100)"=w344) -> ("number"=w340:dbl)  [unwired: 9 in]
              n178 = call-poly <vilib>:"Random Number (Range).vi"("lower bound (0)"=w348, "upper bound (100)"=w347) -> ("number"=w345:dbl)  [unwired: 9 in]
              n179 = local read "next-state-cluster-const"() -> (w355:T1)
              n180 = Bundle By Name(cluster=w355, "next-state"="move", "bypass-confirm"=TRUE, "PDX"=w345, "PDY"=w340, "BarX"=90.0, "BarY"=35.0, "BMA"=45.0, "PDA"=181.0, "bar-note"=w339) -> (w356:T1)
              n181 = Bundle By Name(cluster=w355, "next-state"="nelder-mead") -> (w357:T1)
              n182 = Build Array (concatenate)(w359, w356, w357) -> (w358:T3)
            }
            n183 = Bundle By Name(cluster=w329, "next-state"="diode-scan-center") -> (w330:T1)
            n184 = Build Array (concatenate)(w332, w330) -> (w331:T3)
          }
          frame "setup-IR" {
            # "Pure Beam (PB)\nPDX 266\nPDY 126\nBX 170\nBY 30\nBA 45\nPDA 180"
            # "IR1\nPDX 232\nPDY 119.5\nBX 85\nBY 20\nBA 17.148\nPDA 238\n\nIR2\nPDX 232\nPDY 119.5\nBX 85\nBY 15\nBA 17.148\nPDA 238\n\nIR3\nPDX 232\nPDY 119.5\nBX 85\nBY 32\nBA 17.148\nPDA 238"
            n185 = local read "state-queue"() -> (w372:T3)
            n186 = local read "next-state-cluster-const"() -> (w363:T1)
            n187 = Bundle By Name(cluster=w363, "next-state"="logfile-setup") -> (w364:T1)
            n188 = Build Array (concatenate)(w372, w364) -> (w365:T3)
            n189 = for {
              N: "# IR measurement points" -> [_]
              shift-right: [w466] -> w369
              shift-left: w365 -> [w474]
              shift-right: [w452] -> w370
              shift-left: u32 0 -> [w449]
              i -> [w465]
              # "PB"
              # "IR1"
              n190 = Multiply(x="IR step size", y=w465) -> (x*y=w459:dbl)
              n191 = local read "next-state-cluster-const"() -> (w455:T1)
              n192 = Add(x="IR1 Bar Y start", y=w459) -> (x+y=w445:dbl)
              n193 = Add(x="IR1 Bar X start", y=w459) -> (x+y=w446:dbl)
              n194 = Bundle By Name(cluster=w455, "next-state"="move", "bypass-confirm"=TRUE, "PDX"="IR PDX", "PDY"="IR PDY", "BarX"=w446, "BarY"=w445, "BMA"="IR BMA", "PDA"="IR PDA") -> (w470:T1)
              n195 = Bundle By Name(cluster=w455, "next-state"="move", "bypass-confirm"=TRUE, "PDX"="PB PDX", "PDY"="PB PDY", "BarX"="PB Bar X", "BarY"="PB Bar Y", "BMA"="PB BMA", "PDA"="PB PDA") -> (w454:T1)
              n196 = Increment(x=w449) -> (x+1=w452:u32)
              n197 = Bundle By Name(cluster=w455, "next-state"="nelder-mead", "bar-note"=u8 1, "meas#"=w449) -> (w467:T1)
              n198 = Bundle By Name(cluster=w455, "next-state"="nelder-mead", "bar-note"=u8 0, "meas#"=w449) -> (w453:T1)
              n199 = Build Array (concatenate)(w474, w470, w467, w454, w453) -> (w466:T3)
            }
            n200 = for {
              N: "# IR measurement points" -> [_]
              shift-right: [w434] -> w368
              shift-left: w369 -> [w440]
              shift-right: [w423] -> w367
              shift-left: w370 -> [w420]
              i -> [w433]
              # "PB"
              # "IR2"
              n201 = local read "IR step size"() -> (w413:dbl)
              n202 = local read "IR PDA"() -> (w414:dbl)
              n203 = Multiply(x=w413, y=w433) -> (x*y=w428:dbl)
              n204 = local read "IR PDX"() -> (w417:dbl)
              n205 = local read "IR PDY"() -> (w416:dbl)
              n206 = local read "next-state-cluster-const"() -> (w426:T1)
              n207 = local read "IR BMA"() -> (w415:dbl)
              n208 = Add(x="IR2 BarY start", y=w428) -> (x+y=w418:dbl)
              n209 = Add(x="IR2 BarX start", y=w428) -> (x+y=w419:dbl)
              n210 = local read "PB Bar X"() -> (w409:dbl)
              n211 = local read "PB Bar Y"() -> (w410:dbl)
              n212 = local read "PB BMA"() -> (w408:dbl)
              n213 = local read "PB PDA"() -> (w407:dbl)
              n214 = local read "PB PDX"() -> (w412:dbl)
              n215 = local read "PB PDY"() -> (w411:dbl)
              n216 = Bundle By Name(cluster=w426, "next-state"="move", "bypass-confirm"=TRUE, "PDX"=w417, "PDY"=w416, "BarX"=w419, "BarY"=w418, "BMA"=w415, "PDA"=w414) -> (w436:T1)
              n217 = Bundle By Name(cluster=w426, "next-state"="move", "bypass-confirm"=TRUE, "PDX"=w412, "PDY"=w411, "BarX"=w409, "BarY"=w410, "BMA"=w408, "PDA"=w407) -> (w425:T1)
              n218 = Increment(x=w420) -> (x+1=w423:u32)
              n219 = Bundle By Name(cluster=w426, "next-state"="nelder-mead", "bar-note"=u8 1, "meas#"=w420) -> (w435:T1)
              n220 = Bundle By Name(cluster=w426, "next-state"="nelder-mead", "bar-note"=u8 0, "meas#"=w420) -> (w424:T1)
              n221 = Build Array (concatenate)(w440, w436, w435, w425, w424) -> (w434:T3)
            }
            n222 = for {
              N: "# IR measurement points" -> [_]
              shift-right: [w400] -> w366
              shift-left: w368 -> [w406]
              shift-right: [w389] -> _
              shift-left: w367 -> [w386]
              i -> [w399]
              # "PB"
              # "IR3"
              n223 = local read "IR step size"() -> (w379:dbl)
              n224 = Multiply(x=w379, y=w399) -> (x*y=w394:dbl)
              n225 = local read "IR PDA"() -> (w380:dbl)
              n226 = local read "IR PDX"() -> (w383:dbl)
              n227 = local read "IR PDY"() -> (w382:dbl)
              n228 = local read "next-state-cluster-const"() -> (w392:T1)
              n229 = Add(x="IR3 BarY start", y=w394) -> (x+y=w384:dbl)
              n230 = Add(x="IR3 BarX start", y=w394) -> (x+y=w385:dbl)
              n231 = local read "IR BMA"() -> (w381:dbl)
              n232 = local read "PB Bar X"() -> (w376:dbl)
              n233 = local read "PB Bar Y"() -> (w375:dbl)
              n234 = local read "PB BMA"() -> (w374:dbl)
              n235 = local read "PB PDA"() -> (w373:dbl)
              n236 = local read "PB PDX"() -> (w378:dbl)
              n237 = local read "PB PDY"() -> (w377:dbl)
              n238 = Bundle By Name(cluster=w392, "next-state"="move", "bypass-confirm"=TRUE, "PDX"=w383, "PDY"=w382, "BarX"=w385, "BarY"=w384, "BMA"=w381, "PDA"=w380) -> (w402:T1)
              n239 = Bundle By Name(cluster=w392, "next-state"="move", "bypass-confirm"=TRUE, "PDX"=w378, "PDY"=w377, "BarX"=w376, "BarY"=w375, "BMA"=w374, "PDA"=w373) -> (w391:T1)
              n240 = Increment(x=w386) -> (x+1=w389:u32)
              n241 = Bundle By Name(cluster=w392, "next-state"="nelder-mead", "bar-note"=u8 1, "meas#"=w386) -> (w401:T1)
              n242 = Bundle By Name(cluster=w392, "next-state"="nelder-mead", "bar-note"=u8 0, "meas#"=w386) -> (w390:T1)
              n243 = Build Array (concatenate)(w406, w402, w401, w391, w390) -> (w400:T3)
            }
          }
          frame "setup-BA" {
            # "Pure Beam (PB)\nPDX 266\nPDY 126\nBX 170\nBY 30\nBA 45\nPDA 180"
            # "BA1\nPDX 268\nPDY 126\nBX 229\nBY 30\nBA 45\nPDA 180\n\nBA2\nPDX 268\nPDY 126\nBX 229\nBY 15\nBA 45\nPDA 180\n\nBA3\nPDX 268\nPDY 126\nBX 229\nBY 20\nBA 45\nPDA 180"
            n244 = local read "state-queue"() -> (w486:T3)
            n245 = local read "next-state-cluster-const"() -> (w477:T1)
            n246 = Bundle By Name(cluster=w477, "next-state"="logfile-setup") -> (w478:T1)
            n247 = Build Array (concatenate)(w486, w478) -> (w479:T3)
            n248 = for {
              N: "# BA measurement points" -> [_]
              shift-right: [w580] -> w484
              shift-left: w479 -> [w588]
              shift-right: [w566] -> w482
              shift-left: u32 0 -> [w563]
              i -> [w579]
              # "PB"
              # "BA1"
              n249 = Multiply(x="BA step size", y=w579) -> (x*y=w573:dbl)
              n250 = local read "next-state-cluster-const"() -> (w569:T1)
              n251 = Add(x="BA1 Bar Y start", y=w573) -> (x+y=w559:dbl)
              n252 = Add(x="BA1 BarX start", y=w573) -> (x+y=w560:dbl)
              n253 = Bundle By Name(cluster=w569, "next-state"="move", "bypass-confirm"=TRUE, "PDX"="BA PDX", "PDY"="BA PDY", "BarX"=w560, "BarY"=w559, "BMA"="BA BMA", "PDA"="BA PDA") -> (w584:T1)
              n254 = Bundle By Name(cluster=w569, "next-state"="move", "bypass-confirm"=TRUE, "PDX"=266.0 ("BarX"), "PDY"=126.0 ("BarY"), "BarX"=170.0 ("x"), "BarY"=30.0 ("x"), "BMA"=45.0, "PDA"=180.0) -> (w568:T1)
              n255 = Increment(x=w563) -> (x+1=w566:u32)
              n256 = Bundle By Name(cluster=w569, "next-state"="nelder-mead", "bar-note"=u8 2, "meas#"=w563) -> (w581:T1)
              n257 = Bundle By Name(cluster=w569, "next-state"="nelder-mead", "bar-note"=u8 0, "meas#"=w563) -> (w567:T1)
              n258 = Build Array (concatenate)(w588, w584, w581, w568, w567) -> (w580:T3)
            }
            n259 = for {
              N: "# BA measurement points" -> [_]
              shift-right: [w514] -> w483
              shift-left: w484 -> [w520]
              shift-right: [w501] -> w481
              shift-left: w482 -> [w498]
              i -> [w513]
              # "PB"
              # "BA2"
              n260 = local read "BA step size"() -> (w487:dbl)
              n261 = local read "BA BMA"() -> (w489:dbl)
              n262 = local read "BA PDA"() -> (w488:dbl)
              n263 = Multiply(x=w487, y=w513) -> (x*y=w508:dbl)
              n264 = local read "BA PDY"() -> (w490:dbl)
              n265 = local read "BA PDX"() -> (w491:dbl)
              n266 = local read "next-state-cluster-const"() -> (w504:T1)
              n267 = Add(x="BA2 BarY start", y=w508) -> (x+y=w496:dbl)
              n268 = Add(x="BA2 BarX start", y=w508) -> (x+y=w497:dbl)
              n269 = Bundle By Name(cluster=w504, "next-state"="move", "bypass-confirm"=TRUE, "PDX"=w491, "PDY"=w490, "BarX"=w497, "BarY"=w496, "BMA"=w489, "PDA"=w488) -> (w516:T1)
              n270 = Bundle By Name(cluster=w504, "next-state"="move", "bypass-confirm"=TRUE, "PDX"=266.0 ("BarX"), "PDY"=126.0 ("BarY"), "BarX"=170.0 ("x"), "BarY"=30.0 ("x"), "BMA"=45.0, "PDA"=180.0) -> (w503:T1)
              n271 = Increment(x=w498) -> (x+1=w501:u32)
              n272 = Bundle By Name(cluster=w504, "next-state"="nelder-mead", "bar-note"=u8 2, "meas#"=w498) -> (w515:T1)
              n273 = Bundle By Name(cluster=w504, "next-state"="nelder-mead", "bar-note"=u8 0, "meas#"=w498) -> (w502:T1)
              n274 = Build Array (concatenate)(w520, w516, w515, w503, w502) -> (w514:T3)
            }
            n275 = for {
              N: "# BA measurement points" -> [_]
              shift-right: [w548] -> w480
              shift-left: w483 -> [w554]
              shift-right: [w535] -> _
              shift-left: w481 -> [w532]
              i -> [w547]
              # "PB"
              # "BA3"
              n276 = local read "BA step size"() -> (w521:dbl)
              n277 = local read "BA BMA"() -> (w525:dbl)
              n278 = local read "BA PDA"() -> (w524:dbl)
              n279 = Multiply(x=w521, y=w547) -> (x*y=w542:dbl)
              n280 = local read "BA PDY"() -> (w522:dbl)
              n281 = local read "BA PDX"() -> (w523:dbl)
              n282 = local read "next-state-cluster-const"() -> (w538:T1)
              n283 = Add(x="BA3 BarY start", y=w542) -> (x+y=w530:dbl)
              n284 = Add(x="BA3 BarX start", y=w542) -> (x+y=w531:dbl)
              n285 = Bundle By Name(cluster=w538, "next-state"="move", "bypass-confirm"=TRUE, "PDX"=w523, "PDY"=w522, "BarX"=w531, "BarY"=w530, "BMA"=w525, "PDA"=w524) -> (w550:T1)
              n286 = Bundle By Name(cluster=w538, "next-state"="move", "bypass-confirm"=TRUE, "PDX"=266.0 ("BarX"), "PDY"=126.0 ("BarY"), "BarX"=170.0 ("x"), "BarY"=30.0 ("x"), "BMA"=45.0, "PDA"=180.0) -> (w537:T1)
              n287 = Increment(x=w532) -> (x+1=w535:u32)
              n288 = Bundle By Name(cluster=w538, "next-state"="nelder-mead", "bar-note"=u8 2, "meas#"=w532) -> (w549:T1)
              n289 = Bundle By Name(cluster=w538, "next-state"="nelder-mead", "bar-note"=u8 0, "meas#"=w532) -> (w536:T1)
              n290 = Build Array (concatenate)(w554, w550, w549, w537, w536) -> (w548:T3)
            }
          }
          frame "logfile-setup" {
            n291 = local read "log-path"() -> (w594:path)
            n292 = Path To String(path=w594) -> (string=w592:string)
            n293 = Concatenate Strings("Use logfile set at program start or start new file? \n\nLogfile set at start:\n", w592) -> (w591:string)
            n294 = Two Button Dialog(message=w591, 1:"Continue" ("F button name (\"Cancel\")"), 2:"Make New File" ("T button name (\"OK\")")) -> (T button?=w595:bool)
            n295 = case shown="True" w595 {
              frame False {
              }
              frame True {
                w599 = FALSE  # dev-mode
                n296 = call "log_file_setup.vi"("dev-mode"=w599) -> ("error out"=w597:errorcluster, "appended path"=w598:path)  [unwired: 8 in, 1 out]
                n297 = local write "log-path"(w598) -> ()
                n298 = local write "log-error"(w597) -> ()
              }
            }
            n299 = local read "state-queue"() -> (w596:T3)
          }
        }
        n300 = Subtract(x=w93, y=w92) -> (x-y=→"loop-rate":u32)
        n301 = Get Date/Time In Seconds() -> (seconds since 1Jan1904=w88:timestamp)
        n302 = Format Date/Time String(time format string (%c)="%Y-%m-%d %H:%M:%S", seconds (now)=w88) -> (date/time string=→"Current Time:":string)  [unwired: 1 in]
      }
    }
    frame #4 {
      # "Close connection to meter"
      n303 = local read "main-stage-refs"() -> (w601:T2)
      n304 = Unbundle By Name(w601) -> ("Bar X main"=w607:refnum<k24>, "Bar Y main"=w606:refnum<k24>, "PD X main"=w605:refnum<k24>, "PD Y main"=w604:refnum<k24>, "BMA main"=w603:refnum<k24>, "PDA main"=w602:refnum<k24>)
      n305 = local write "start-msg"("Closing Stages" ("String")) -> ()
      n306 = invoke class="BenchtopStepperControl" method="CloseDevice"(reference=w603) -> (error out=w612:errorcluster)  [unwired: 2 in, 2 out]
      n307 = invoke class="BenchtopStepperControl" method="CloseDevice"(reference=w602) -> (error out=w613:errorcluster)  [unwired: 2 in, 2 out]
      n308 = invoke class="LongTravelStageControl" method="CloseDevice"(reference=w607) -> (error out=w608:errorcluster)  [unwired: 2 in, 2 out]
      n309 = invoke class="LongTravelStageControl" method="CloseDevice"(reference=w606) -> (error out=w609:errorcluster)  [unwired: 2 in, 2 out]
      n310 = invoke class="LongTravelStageControl" method="CloseDevice"(reference=w605) -> (error out=w610:errorcluster)  [unwired: 2 in, 2 out]
      n311 = invoke class="LongTravelStageControl" method="CloseDevice"(reference=w604) -> (error out=w611:errorcluster)  [unwired: 2 in, 2 out]
      n312 = local read "stage-error"() -> (w614:errorcluster)
      n313 = Merge Errors(w614, w608, w609, w610, w611, w612, w613) -> (w615:errorcluster)
      n314 = local write "stage-error"(w615) -> ()
    }
    frame #5 {
      # "Section deletes log file if nothing is written to it\nto prevent just a ton of empty files during development"
      n315 = local read "log-error"() -> (w620:errorcluster)
      n316 = local read "keep-file"() -> (w618:bool)
      n317 = local read "log-path"() -> (w619:path)
      n318 = case shown="False" w618 {
        tunnel: w620 -> [w623 w625]
        tunnel: [w624 w625] -> w621
        tunnel: w619 -> [w622 _]
        frame False {
          n319 = Delete(path (use dialog)=w622, error in=w623) -> (error out=w624:errorcluster)  [unwired: 3 in, 2 out]
        }
        frame True {
        }
      }
      n320 = local write "start-msg"("Program Stopped" ("String")) -> ()
      n321 = local write "Just Measure"(FALSE ("Just Measure")) -> ()
      n322 = local write "log-error"(w621) -> ()
    }
  }
